vi "calculate f comp.vi"(11 "Matriz m\nobservada":T1) -> (2 "Componente \nde n_o em f":T1, 3 "<f,m_o>/|f|^2":dbl format="%.2f", 4 "error":i32)   [LabVIEW 2018]
uses:
  <vilib>/Analysis/Matrix/Datatypes/RealMatrix.ctl
  <vilib>/Analysis/_algsub.llb/Real Vector Norm.vi
  <vilib>/Analysis/baseanly.llb/Real Dot Product.vi
  <vilib>/Analysis/Matrix/Numeric/Conversions/Array To Matrix - RA.vi
  <vilib>/Analysis/NI_AALBase.lvlib
  <vilib>/Analysis/Matrix/NI_Matrix.lvlib
  <vilib>/Analysis/NI_AALPro.lvlib
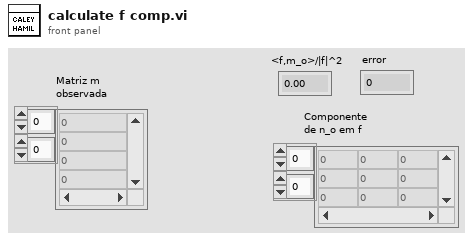
[diagram p1: front panel]
types:
  T1 = typedef "NI_Matrix.lvlib/RealMatrix.ctl" = dbl[][]
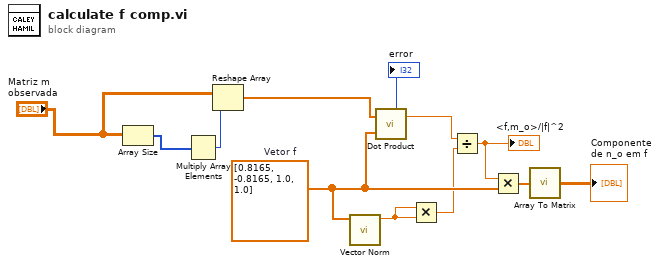
[diagram p0: block diagram]
diagram:
  w10 = dbl[] [0.8165, -0.8165, 1.0, 1.0]  # Vetor f
  n1 = Array Size(array="Matriz m\nobservada") -> (size(s)=w4:i32[])
  n2 = Multiply Array Elements(1:w4) -> (0:w3:i32)
  n3 = Reshape Array("Matriz m\nobservada", w3) -> (w1:dbl[])
  n4 = call-poly <vilib>:"Vector Norm.vi"("Input Vector"=w10) -> ("norm"=w8:dbl)  [unwired: 9 in, 1 out]
  n5 = call-poly <vilib>:"Dot Product.vi"("Y Vector"=w10, "X Vector"=w1) -> ("error"=→"error":i32, "X * Y"=w9:dbl)
  n6 = Multiply(x=w8, y=w8) -> (x*y=w7:dbl)
  n7 = Divide(x=w9, y=w7) -> (x/y=w6:dbl)
  "<f,m_o>/|f|^2" <- w6
  n8 = Multiply(x=w6, y=w10) -> (x*y=w11:dbl[])
  n9 = call-poly <vilib>:"Array To Matrix.vi"("Real 1D Array"=w11) -> ("Real Matrix (Column Vector)"=→"Componente \nde n_o em f":T1)
